vi "Object Array Replace.vi"() -> ()   [LabVIEW 2016]
uses:
  Classes/Runtime/Transfer/Runtime.Transfer.lvclass
  Typedefs/Transfer Direction.ctl
  Classes/Runtime/Channel/Runtime.Channel.lvclass
  Classes/Runtime/Transfer/Properties/Write direction.vi
  Classes/Runtime/Transfer/Properties/Write byte order.vi
  Classes/Runtime/Transfer/Properties/Write Channel Runtimes.vi
  APIs/Runtime/Get Object Size (Channel).vi
  Data Sharing Framework.Configuration.lvlib
  APIs/Runtime/Data Sharing Framework.Runtime.lvlib
panel:
  out "size":i32
  out "object size":i32
  out "array size":i32
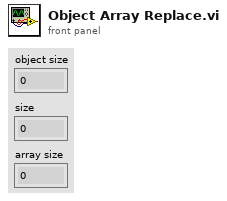
[diagram p1: front panel]
types:
  T1 = enum16{"big-endian, network order", "native, host order", "little-endian"}
  T2 = typedef "Data Sharing Framework.Configuration.lvlib/Transfer Direction.ctl" = enum16{"Tx", "Rx"}
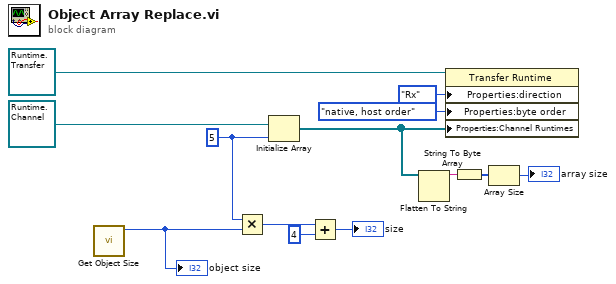
[diagram p0: block diagram]
diagram:
  w5 = 5 ("dimension size")
  n1 = call-poly "Get Object Size.vi"() -> ("size"=w1:u64)  [unwired: 10 in, 1 out]
  "object size" <- w1
  n2 = Multiply(x=w5, y=w1) -> (x*y=w4:u64)
  n3 = Initialize Array(refnum<class "Runtime.Channel.lvclass"> refnum ("Data Sharing Framework.Runtime.lvlib:Channel Runtime"), w5) -> (w3:refnum<class "Runtime.Channel.lvclass">[])
  n4 = Add(x=w4, y=4) -> (x+y=→"size":u64)
  n5 = Flatten To String(anything=w3) -> (data string=w8:string)  [unwired: 3 in, 2 out]
  n6 = property class="Transfer Runtime"(reference=refnum<class "Runtime.Transfer.lvclass"> refnum ("Data Sharing Framework.Runtime.lvlib:Transfer Runtime"), "Properties:direction"=Transfer_Direction."Rx" ("direction"), "Properties:byte order"=T1."native, host order" ("byte order"), "Properties:Channel Runtimes"=w3) -> ()  [unwired: 1 in, 2 out]
  n7 = String To Byte Array(string=w8) -> (unsigned byte array=w9:u8[])
  n8 = Array Size(array=w9) -> (size(s)=→"array size":i32)
